vi "Periodic Tasks.vi"(8 "error in":errorcluster) -> ()   [LabVIEW 2017]
doc: "This VI runs in parallel to other tasks. It can contain as many user-defined periodic loops as you need. These can carry out PID or other sorts of timed response."
uses:
  Public/Documents/Cross The Road Electronics/Phoenix-LabVIEW/Motor Controller/Controls/CTRE_Phoenix_MotorControl_FeedbackDevice.ctl
  Public/Documents/Cross The Road Electronics/Phoenix-LabVIEW/Motor Controller/Controls/CTRE_Phoenix_MotorControl_StatusFrameEnhanced.ctl
  Public/Documents/Cross The Road Electronics/Phoenix-LabVIEW/Motor Controller/Controls/CTRE_Phoenix_MotorControl_ControlMode.ctl
  Public/Documents/Cross The Road Electronics/Phoenix-LabVIEW/Motor Controller/Controls/CTRE_Phoenix_MotorControl_TrajectoryPointTimeDur.ctl
  <vilib>/Rock Robotics/WPI/Utilities/WPI_GetSetVariantRefNum.vi
  <vilib>/Utility/file.llb/Read Delimited Spreadsheet (DBL).vi
panel:
  out "Loop Time":u32
  out "Points in the CSV":i32
  out "Mot Prof Active Position":dbl
  out "Mot Prof Active Velocity":dbl
  out "Mot Prof Count":i32
  out "Mot Prof Active Is Valid":bool
  out "Mot Prof Active Is Last":bool
  out "Mot Prof  Has Under Run":bool
  out "Mot Prof  Is Under Run":bool
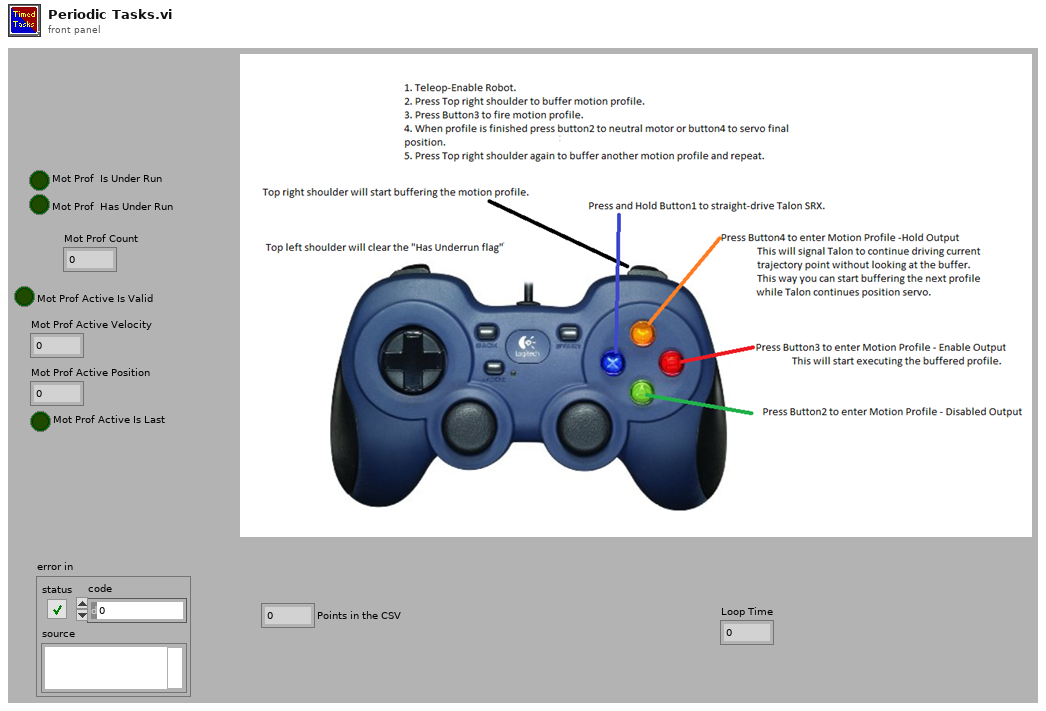
[diagram p1: front panel]
types:
  T1 = typedef "CTRE_Phoenix_MotorControl_StatusFrameEnhanced.ctl" = u16
  T2 = typedef "CTRE_Phoenix_MotorControl_FeedbackDevice.ctl" = i8
  T3 = typedef "WPI_MotorControlDeviceRef.ctl" = cluster{"DeviceStatus":errorcluster, "Type":T4, "PWM":cluster{"PWM Channel":T5, "DeadBand":T6}, "CAN":cluster{"Device Number":u8, "SetOutput VI Ref":variant, "GetOutput VI Ref":variant, "Enable VI Ref":variant, "Disable VI Ref":variant, "Data":variant}, "Invert":bool, "DIO PWM":cluster{"PWM \"Enable\" Channel":T5, "DIOChannel":T7, "PWM Rate":dbl}}
  T4 = typedef "WPI_MotorControlType.ctl" = enum16{"PWM", "CAN", "DIO PWM"}
  T5 = typedef "FPGA_DIOPWMChannel.ctl" = enum8{"PWM 0", "PWM 1", "PWM 2", "PWM 3", "PWM 4", "PWM 5", "PWM 6", "PWM 7", "PWM 8", "PWM 9", "PWM MXP 0", "PWM MXP 1", "PWM MXP 2", "PWM MXP 3", "PWM MXP 4", "PWM MXP 5", "PWM MXP 6", "PWM MXP 7", "PWM MXP 8", "PWM MXP 9", "Invalid"}
  T6 = typedef "WPI_PWMDeadband.ctl" = cluster{"Name":string, "maxPositivePwm":i32, "minPositivePwm":i32, "centerPwm":i32, "maxNegativePwm":i32, "minNegativePwm":i32, "angularRange":u16}
  T7 = typedef "FPGA_DIOChannel.ctl" = enum8{"DIO 0", "DIO 1", "DIO 2", "DIO 3", "DIO 4", "DIO 5", "DIO 6", "DIO 7", "DIO 8", "DIO 9", "DIO MXP 0", "DIO MXP 1", "DIO MXP 2", "DIO MXP 3", "DIO MXP 4", "DIO MXP 5", "DIO MXP 6", "DIO MXP 7", "DIO MXP 8", "DIO MXP 9", "DIO MXP 10", "DIO MXP 11", "DIO MXP 12", "DIO MXP 13", "DIO MXP 14", "DIO MXP 15", "SPI Port CS1", "SPI Port CS2", "SPI Port CS3", "SPI Port MISO", "SPI Port MOSI", "Invalid"}
  T8 = typedef "WPI_JoystickDevRef.ctl" = cluster{"Device":T9}
  T9 = typedef "WPI_JoystickDeviceEnum.ctl" = enum16{"USB 0", "USB 1", "USB 2", "USB 3", "USB 4", "USB 5"}
  T10 = typedef "CTRE_Phoenix_MotorControl_ControlMode.ctl" = u16
  T11 = cluster{"Top Buffer Remaining":i32, "Top Buffer Count":i32, "Bottom Buffer Count":i32, "Has Underrun?":bool, "Is Underrun?":bool, "Active Point Valid?":bool, "Is Last?":bool, "Profile Slot Select 0":i32, "Output Enable":i32, "Time Duration (ms)":i32, "Profile Slot Select 1":i32}
  T12 = typedef "CTRE_Phoenix_MotorControl_TrajectoryPointTimeDur.ctl" = i32
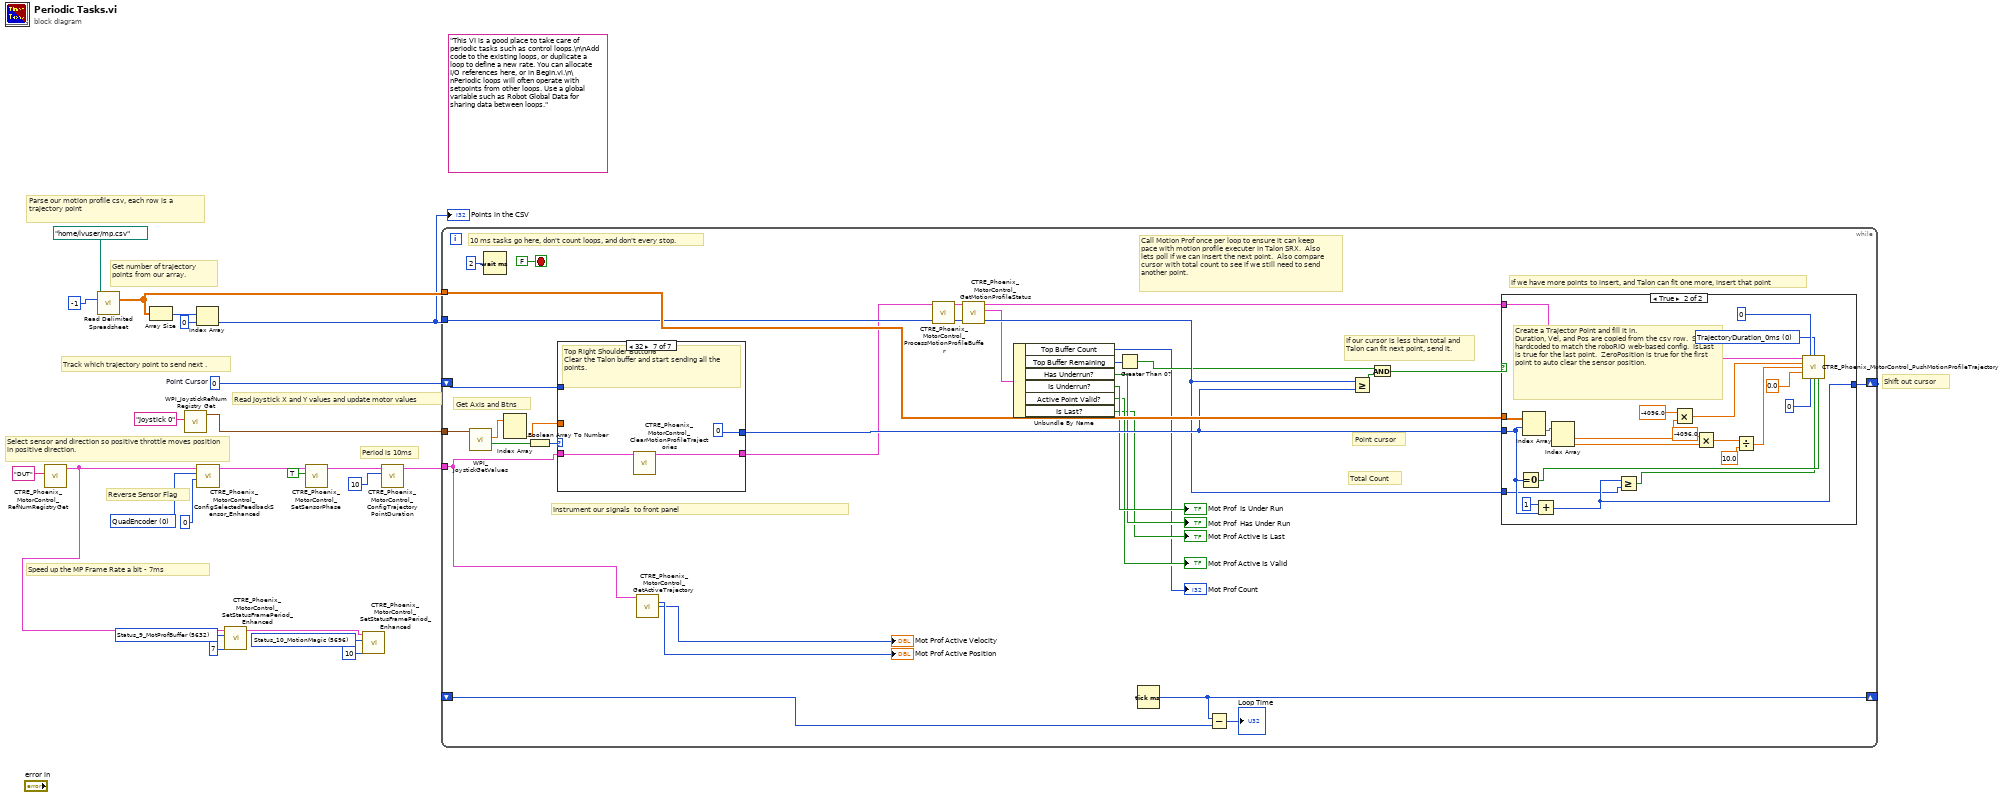
[diagram p0: block diagram]
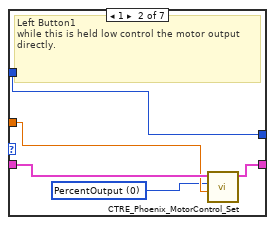
[diagram p3: hidden frame]
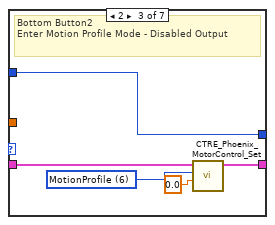
[diagram p4: hidden frame]
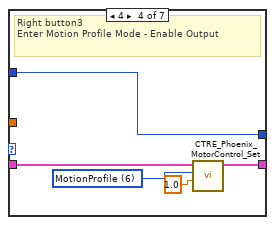
[diagram p5: hidden frame]
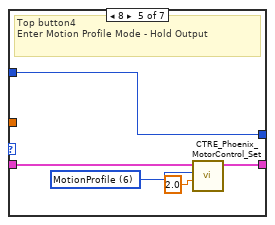
[diagram p6: hidden frame]
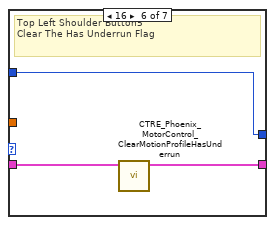
[diagram p7: hidden frame]
diagram:
  w6 = T1 5696 items=["Status_1_General"=5120, "Status_2_Feedback0"=5184, "Status_3_Quadrature"=5248, "Status_4_AinTempVbat"=5312, "Status_6_Misc"=5440, "Status_7_CommStatus"=5504, "Status_8_PulseWidth"=5568, "Status_9_MotProfBuffer"=5632, "Status_10_MotionMagic"=5696, "Status_11_UartGadgeteer"=5760, "Status_12_Feedback1"=5824, "Status_13_Base_PIDF0"=5888, "Status_14_Turn_PIDF1"=5952, "Status_15_FirmwareApiStatus"=6016] ("Status Frame")
  w11 = T1 5632 items=["Status_1_General"=5120, "Status_2_Feedback0"=5184, "Status_3_Quadrature"=5248, "Status_4_AinTempVbat"=5312, "Status_6_Misc"=5440, "Status_7_CommStatus"=5504, "Status_8_PulseWidth"=5568, "Status_9_MotProfBuffer"=5632, "Status_10_MotionMagic"=5696, "Status_11_UartGadgeteer"=5760, "Status_12_Feedback1"=5824, "Status_13_Base_PIDF0"=5888, "Status_14_Turn_PIDF1"=5952, "Status_15_FirmwareApiStatus"=6016] ("Status Frame")
  w13 = T2 0 items=["None"=-1, "QuadEncoder"=0, "Analog"=2, "Tachometer"=4, "Pulse Width Encoded Position"=8, "Sensor Sum (S0 + S1)"=9, "Sensor Difference (D0 - D1)"=10, "Remote Source 0"=11, "Remote Source 1"=12, "Software Emulated"=15] ("Feedback Device")
  w18 = 0  # Point Cursor
  (unwired) "This VI is a good place to take care of periodic tasks such as control loops.\n\nAdd code to the existing loops, or duplicate a loop to define a new rate. You can allocate I/O references here, or in Begin.vi.\n\nPeriodic loops will often operate with setpoints from other loops. Use a global variable such as Robot Global Data for sharing data between loops."
  # "Period is 10ms"
  # "Shift out cursor"
  # "Read Joystick X and Y values and update motor values"
  # "Reverse Sensor Flag"
  # "Select sensor and direction so positive throttle moves position in positive direction."
  # "Get number of trajectory points from our array."
  # "Track which trajectory point to send next ."
  # "Speed up the MP Frame Rate a bit - 7ms"
  # "Parse our motion profile csv, each row is a trajectory point"
  n1 = call "CTRE_Phoenix_MotorControl_RefNumRegistryGet.vi"("refnum name"="DUT") -> ("PhoenixMotorControlDevRef"=w9:T3)  [unwired: 9 in, 1 out]
  n2 = call-poly <vilib>:"Read Delimited Spreadsheet.vi"("file path (dialog if empty)"=path "/home/lvuser/mp.csv" ("file path (use dialog)"), "number of rows (all:-1)"=-1) -> ("all rows"=w15:dbl[][])  [unwired: 8 in, 5 out]
  n3 = Array Size(array=w15) -> (size(s)=w16:i32[])
  n4 = call <vilib>:"WPI_JoystickRefNum Registry Get.vi"("refnum name"="Joystick 0") -> ("JoystickDevRef"=w21:T8)  [unwired: 1 in, 9 out]
  n5 = Index Array(array=w16, index=0) -> (element=w14:i32)
  "Points in the CSV" <- w14
  n6 = call "CTRE_Phoenix_MotorControl_ConfigSelectedFeedbackSensor_Enhanced.vi"("pidLoopIdx"=0, "Feedback Device"=w13, "PhoenixMotorControlDevRef"=w9) -> ("PhoenixMotorControlDevRef"=w8:T3)  [unwired: 7 in, 1 out]
  n7 = call "CTRE_Phoenix_MotorControl_SetStatusFramePeriod_Enhanced.vi"("periodMs"=7, "Status Frame"=w11, "PhoenixMotorControlDevRef"=w9) -> ("PhoenixMotorControlDevRef"=w4:T3)  [unwired: 7 in, 1 out]
  n8 = call "CTRE_Phoenix_MotorControl_SetSensorPhase.vi"("PhaseSensor"=TRUE, "PhoenixMotorControlDevRef"=w8) -> ("PhoenixMotorControlDevRef"=w1:T3)  [unwired: 8 in, 1 out]
  n9 = call "CTRE_Phoenix_MotorControl_SetStatusFramePeriod_Enhanced.vi"("periodMs"=10, "Status Frame"=w6, "PhoenixMotorControlDevRef"=w4) -> ()  [unwired: 7 in, 2 out]
  n10 = call "CTRE_Phoenix_MotorControl_ConfigTrajectoryPointDuration.vi"("durationMs"=10 ("periodMs"), "PhoenixMotorControlDevRef"=w1) -> ("PhoenixMotorControlDevRef"=w2:T3)  [unwired: 8 in, 1 out]
  n11 = while {
    tunnel: w21 -> [w52]
    tunnel: w15 -> [w51]
    shift-right: [w50] -> _
    shift-left: w18 -> [w49]
    tunnel: w14 -> [w46]
    tunnel: w2 -> [w24]
    shift-right: [w27] -> _
    shift-left: _ -> [w26]
    stop <- FALSE stop-if-true
    # "Call Motion Prof once per loop to ensure it can keep pace with motion profile executer in Talon SRX.  Also lets poll if we can insert the next point.  Also compare cursor with total count to see if we still need to send another point."
    # "Instrument our signals  to front panel"
    # "Get Axis and Btns"
    # "Point cursor"
    # "Total Count"
    # "If our cursor is less than total and Talon can fit next point, send it."
    # "If we have more points to insert, and Talon can fit one more, insert that point"
    # "10 ms tasks go here, don't count loops, and don't every stop."
    n12 = call <vilib>:"WPI_JoystickGetValues.vi"("JoystickDevRef"=w52) -> ("Buttons"=w40:bool[], "Axes"=w41:dbl[])  [unwired: 6 in, 3 out]
    n13 = Wait (ms)(milliseconds to wait=u32 2) -> ()  [unwired: 1 out]
    n14 = Index Array(array=w41) -> (element #2=w38:dbl)  [unwired: 2 in, 1 out]
    n15 = Boolean Array To Number(Boolean array=w40) -> (number=w39:u32)
    n16 = case shown="32" w39 {
      tunnel: w24 -> [w56 w61 w64 w69 w76 w77 w80]
      tunnel: [w56 w60 w63 w68 w73 w78 w81] -> w44
      tunnel: w38 -> [_ w59 _ _ _ _ _]
      tunnel: [w55 w58 w62 w67 w72 w79 0 ("Capacity")] -> w47
      tunnel: w49 -> [w55 w58 w62 w67 w72 w79 _]
      frame Default {
        # "No buttons we care about"
      }
      frame 1 {
        w57 = T10 0 items=["PercentOutput"=0, "Position"=1, "Velocity"=2, "Current"=3, "Follower"=5, "MotionProfile"=6, "MotionMagic"=7, "MotionMagicArc"=8, "MotionProfileArc"=10, "Disabled"=15] ("Control Mode")
        # "Left Button1\nwhile this is held low control the motor output directly."
        n17 = call "CTRE_Phoenix_MotorControl_Set.vi"("Output"=w59, "Control Mode"=w57, "PhoenixMotorControlDevRef"=w61) -> ("PhoenixMotorControlDevRef"=w60:T3)  [unwired: 7 in, 1 out]
      }
      frame 2 {
        w66 = T10 6 items=["PercentOutput"=0, "Position"=1, "Velocity"=2, "Current"=3, "Follower"=5, "MotionProfile"=6, "MotionMagic"=7, "MotionMagicArc"=8, "MotionProfileArc"=10, "Disabled"=15] ("Control Mode")
        # "Bottom Button2\nEnter Motion Profile Mode - Disabled Output"
        n18 = call "CTRE_Phoenix_MotorControl_Set.vi"("Output"=0.0, "Control Mode"=w66, "PhoenixMotorControlDevRef"=w64) -> ("PhoenixMotorControlDevRef"=w63:T3)  [unwired: 7 in, 1 out]
      }
      frame 4 {
        w71 = T10 6 items=["PercentOutput"=0, "Position"=1, "Velocity"=2, "Current"=3, "Follower"=5, "MotionProfile"=6, "MotionMagic"=7, "MotionMagicArc"=8, "MotionProfileArc"=10, "Disabled"=15] ("Control Mode")
        # "Right button3\nEnter Motion Profile Mode - Enable Output"
        n19 = call "CTRE_Phoenix_MotorControl_Set.vi"("Output"=1.0, "Control Mode"=w71, "PhoenixMotorControlDevRef"=w69) -> ("PhoenixMotorControlDevRef"=w68:T3)  [unwired: 7 in, 1 out]
      }
      frame 8 {
        w75 = T10 6 items=["PercentOutput"=0, "Position"=1, "Velocity"=2, "Current"=3, "Follower"=5, "MotionProfile"=6, "MotionMagic"=7, "MotionMagicArc"=8, "MotionProfileArc"=10, "Disabled"=15] ("Control Mode")
        # "Top button4\nEnter Motion Profile Mode - Hold Output"
        n20 = call "CTRE_Phoenix_MotorControl_Set.vi"("Output"=2.0, "Control Mode"=w75, "PhoenixMotorControlDevRef"=w76) -> ("PhoenixMotorControlDevRef"=w73:T3)  [unwired: 7 in, 1 out]
      }
      frame 16 {
        # "Top Left Shoulder Button5\nClear The Has Underrun Flag"
        n21 = call "CTRE_Phoenix_MotorControl_ClearMotionProfileHasUnderrun.vi"("PhoenixMotorControlDevRef"=w77) -> ("PhoenixMotorControlDevRef"=w78:T3)  [unwired: 9 in, 1 out]
      }
      frame 32 {
        # "Top Right Shoulder Button6\nClear the Talon buffer and start sending all the points."
        n22 = call "CTRE_Phoenix_MotorControl_ClearMotionProfileTrajectories.vi"("PhoenixMotorControlDevRef"=w80) -> ("PhoenixMotorControlDevRef"=w81:T3)  [unwired: 13 in, 1 out]
      }
    }
    n23 = call "CTRE_Phoenix_MotorControl_GetActiveTrajectory.vi"("PhoenixMotorControlDevRef"=w24) -> ("Position (Sensor Units)"=→"Mot Prof Active Position":i32, "Velocity (Sensor Units per 100 ms)"=→"Mot Prof Active Velocity":i32)  [unwired: 10 in, 3 out]
    n24 = call "CTRE_Phoenix_MotorControl_ProcessMotionProfileBuffer.vi"("PhoenixMotorControlDevRef"=w44) -> ("PhoenixMotorControlDevRef"=w35:T3)  [unwired: 13 in, 1 out]
    n25 = call "CTRE_Phoenix_MotorControl_GetMotionProfileStatus.vi"("PhoenixMotorControlDevRef"=w35) -> ("Motion Profile Status"=w37:T11, "PhoenixMotorControlDevRef"=w43:T3)  [unwired: 8 in, 1 out]
    n26 = Unbundle By Name(w37) -> ("Top Buffer Count"=→"Mot Prof Count":i32, "Top Buffer Remaining"=w36:i32, "Has Underrun?"=→"Mot Prof  Has Under Run":bool, "Is Underrun?"=→"Mot Prof  Is Under Run":bool, "Active Point Valid?"=→"Mot Prof Active Is Valid":bool, "Is Last?"=→"Mot Prof Active Is Last":bool)
    n27 = Greater Than 0?(x=w36) -> (x > 0?=w42:bool)
    n28 = Tick Count (ms)() -> (millisecond timer value=w27:u32)
    n29 = Subtract(x=w27, y=w26) -> (x-y=→"Loop Time":u32)
    n30 = Greater Or Equal?(x=w46, y=w47) -> (x >= y?=w45:bool)
    n31 = And(x=w42, y=w45) -> (x .and. y?=w48:bool)
    n32 = case shown="True" w48 {
      tunnel: w51 -> [_ w104]
      tunnel: [w83 w100] -> w50
      tunnel: w47 -> [w83 w101]
      tunnel: w46 -> [_ w99]
      tunnel: w43 -> [_ w98]
      frame False {
      }
      frame True {
        w84 = T12 0 items=["TrajectoryDuration_0ms"=0, "TrajectoryDuration_5ms"=5, "TrajectoryDuration_10ms"=10, "TrajectoryDuration_20ms"=20, "TrajectoryDuration_30ms"=30, "TrajectoryDuration_40ms"=40, "TrajectoryDuration_50ms"=50, "TrajectoryDuration_100ms"=100] ("durationMs")
        # "Create a Trajector Point and fill it in.\nDuration, Vel, and Pos are copied from the csv row.  Slot is hardcoded to match the roboRIO web-based config.  IsLast is true for the last point.  ZeroPosition is true for the first point to auto clear the sensor position."
        n33 = Equal To 0?(x=w101) -> (x = 0?=w96:bool)
        n34 = Index Array(array=w104, index (row)=w101) -> (element=w102:dbl[])  [unwired: 1 in]
        n35 = Add(x=u32 1, y=w101) -> (x+y=w100:u32)
        n36 = Index Array(array=w102) -> (element #1=w92:dbl, element #2=w89:dbl)  [unwired: 2 in]
        n37 = Greater Or Equal?(x=w100, y=w99) -> (x >= y?=w95:bool)
        n38 = Multiply(x=-4096.0, y=w92) -> (x*y=w91:dbl)
        n39 = Multiply(x=-4096.0, y=w89) -> (x*y=w87:dbl)
        n40 = Divide(x=w87, y=10.0) -> (x/y=w85:dbl)
        n41 = call "CTRE_Phoenix_MotorControl_PushMotionProfileTrajectory.vi"("PhoenixMotorControlDevRef"=w98, "profileSlotSelect1"=0, "durationMs"=w84, "position"=w91, "velocity"=w85, "headingDeg"=0.0, "profileSlotSelect0"=0, "isLastPoint?"=w95, "Zero Position?"=w96) -> ()  [unwired: 5 in, 2 out]
      }
    }
  }
